vi "restart_acquire_sequence.vi"(8 "error in":errorcluster, 11 "Queue in":refnum<queue>) -> (0 "error out":errorcluster, 3 "queue out":refnum<queue>)   [LabVIEW 2012]
uses:
  typedefs/MicroscopeEvent.ctl
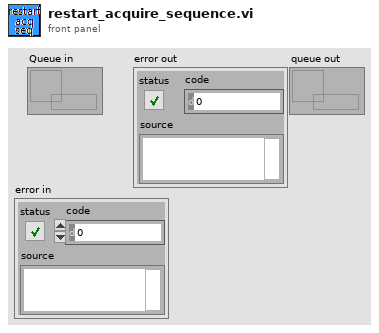
[diagram p1: front panel]
types:
  T1 = typedef "MicroscopeEvent.ctl" = enum16{"M.Wait", "M.RunRotation", "M.Flush", "M.Init", "M.InitStage", "M.InitImageData", "M.ReinitImageData", "M.ReinitImageParams", "M.GetSetParams", "M.InitFastHardware", "M.Pre-Acquire", "M.Acquire", "M.PostAcquire", "M.StopAcquire", "M.SetAcqStatusTrue", "M.SetAcqStatusFalse", "M.ClearImageData", "M.MoveStageDiscrete", "M.MoveStageToTarget1", "M.MoveStageToTarget2", "M.MoveStageToTarget3", "M.OpenShutters", "M.CloseShutters", "M.StartAcquireSequence", "M.ChangeParameters", "M.OpenStokes", "M.OpenPump", "M.RunSW"}
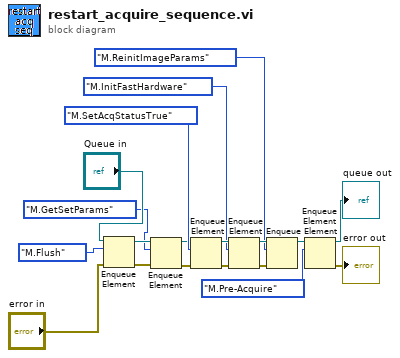
[diagram p0: block diagram]
diagram:
  n1 = Enqueue Element(queue="Queue in", element=MicroscopeEvent."M.Flush", error in (no error)="error in") -> (queue out=w4:refnum<queue>, error out=w5:errorcluster)  [unwired: 1 in, 1 out]
  n2 = Enqueue Element(queue=w4, element=MicroscopeEvent."M.GetSetParams", error in (no error)=w5) -> (queue out=w12:refnum<queue>, error out=w11:errorcluster)  [unwired: 1 in, 1 out]
  n3 = Enqueue Element(queue=w12, element=MicroscopeEvent."M.SetAcqStatusTrue", error in (no error)=w11) -> (queue out=w19:refnum<queue>, error out=w14:errorcluster)  [unwired: 1 in, 1 out]
  n4 = Enqueue Element(queue=w19, element=MicroscopeEvent."M.InitFastHardware" ("t"), error in (no error)=w14) -> (queue out=w10:refnum<queue>, error out=w8:errorcluster)  [unwired: 1 in, 1 out]
  n5 = Enqueue Element(queue=w10, element=MicroscopeEvent."M.ReinitImageParams", error in (no error)=w8) -> (queue out=w9:refnum<queue>)  [unwired: 1 in, 2 out]
  n6 = Enqueue Element(queue=w9, element=MicroscopeEvent."M.Pre-Acquire" ("t")) -> (queue out=→"queue out":refnum<queue>, error out=→"error out":errorcluster)  [unwired: 2 in, 1 out]
